vi "Reverse Bit Order.vi"   [LabVIEW 2016, in "SPIVI.lvlib"]
uses:
  SPIVI.lvlib
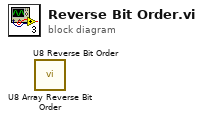
[diagram p0: block diagram]
diagram:
  n1 = call "U8 Array Reverse Bit Order.vi"() -> ()  [unwired: 1 in, 1 out]
  n2 = call "U8 Reverse Bit Order.vi"() -> ()  [unwired: 1 in, 1 out]
